vi "PassOrFail (SubVI).vi"(5 "disabled index (col)":i32, 7 "index (row)":i32, 8 "error in (no error)":errorcluster, 10 "Boolean":bool, 11 "Table in":refnum<vi>) -> (0 "error out":errorcluster)   [LabVIEW 2017]
uses:
  <vilib>/Utility/miscctls.llb/LVRowAndColumnTypeDef.ctl
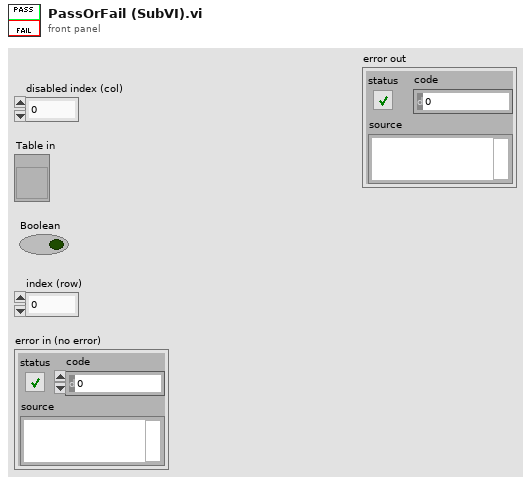
[diagram p1: front panel]
types:
  T1 = typedef "LVRowAndColumnTypeDef.ctl" = cluster{"Row":i32, "Column":i32}
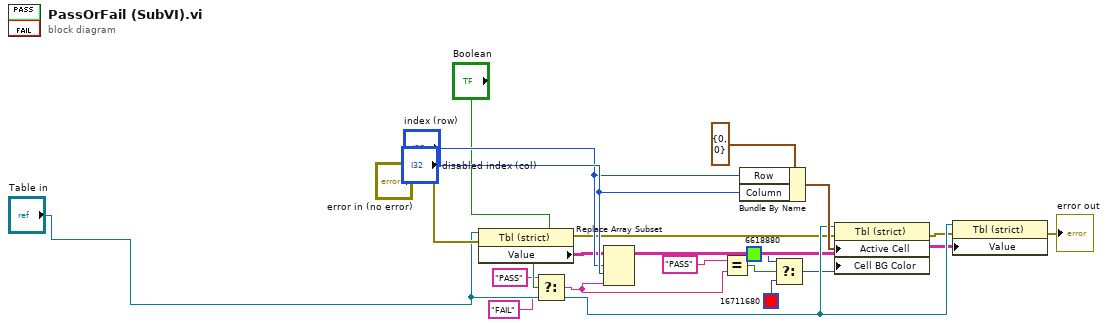
[diagram p0: block diagram]
diagram:
  n1 = property class="Tbl (strict)"(reference="Table in", error in="error in (no error)") -> (error out=w10:errorcluster, "Value"=w7:string[][])  [unwired: 1 out]
  n2 = Select(t="PASS" ("x"), s="Boolean", f="FAIL" ("x")) -> (s? t:f=w13:string)
  n3 = Replace Array Subset(array=w7, new element=w13, index (row)="index (row)", index (col)="disabled index (col)") -> (w8:string[][])
  n4 = Equal?(x="PASS", y=w13) -> (x = y?=w2:bool)
  n5 = Bundle By Name(cluster=T1 {"Row"=0, "Column"=0} ("Active Cell:Active Cell"), "Row"="index (row)", "Column"="disabled index (col)") -> (w18:T1)
  n6 = Select(t=u32 6618880, s=w2, f=u32 16711680) -> (s? t:f=w6:u32)
  n7 = property class="Tbl (strict)"(reference="Table in", error in=w10, "Active Cell"=w18, "Cell BG Color"=w6) -> (error out=w9:errorcluster)  [unwired: 1 out]
  n8 = property class="Tbl (strict)"(reference="Table in", error in=w9, "Value"=w8) -> (error out=→"error out":errorcluster)  [unwired: 1 out]
